vi "ABR-Init Level Series.vi"(0 "Stimulus":T3={"Ear"=enum."Left", "Start (dB)"=20, "Waveform"=enum."TONE PIP", "Stop (dB)"=80, "Frequency (kHz)"=16.0, "Step (dB)"=5, "Rep rate (/sec)"=30.0, "Alternate Polarity"=FALSE} {"Frequency (kHz)" format="%.2f"; "Start (dB)" step=5}, 1 "Data Folder":path, 5 "Runtime In":T1, 9 "Hidden":T2={"AI Samp Rate Hz"=25000.0, "AO Samp Rate Hz"=100000.0, "Duration (ms)"=5.0, "Ramp (ms)"=0.5, "Click width (us)"=0.0, "ITI"=enum."Rate", "Save raw"=FALSE}, 11 "error in (no error)":errorcluster) -> (6 "Runtime Out":T1, 15 "error out":errorcluster)   [LabVIEW 2020]
uses:
  TypeDefs/ABR-Stimulus.ctl
  TypeDefs/ABR-Hidden Params.ctl
  TypeDefs/ABR-Runtime Data.ctl
  epl-vi-lib/Signal Synthesis VIs/Waveform VIs/Pulse Train VIs/Pulse Train Params.ctl
  epl-vi-lib/Signal Synthesis VIs/Waveform VIs/Pulse Train VIs/Pulse Polarity.ctl
  epl-vi-lib/Signal Synthesis VIs/Waveform VIs/Pulse Train VIs/PT-Continuous State.ctl
  epl-vi-lib/Utility VIs/Type Defs/Speaker ring.ctl
panel:
  out "chan index":i32
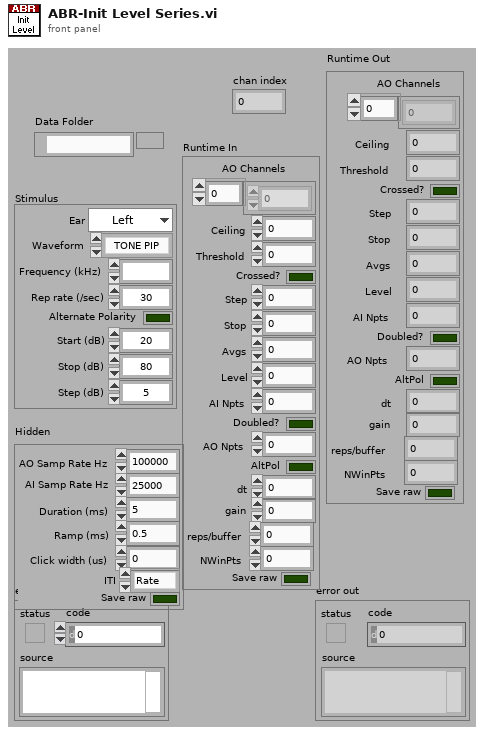
[diagram p1: front panel]
types:
  T1 = typedef "ABR-Runtime Data.ctl" = cluster{"AO Channels":i32[], "Ceiling":dbl, "Threshold":dbl, "Crossed?":bool, "Step":dbl, "Stop":i32, "Avgs":i32, "Level":dbl, "AI Npts":i32, "Doubled?":bool, "AO Npts":i32, "AltPol":bool, "dt":dbl, "gain":dbl, "reps/buffer":i32, "NWinPts":i32, "Save raw":bool}
  T2 = typedef "ABR-Hidden Params.ctl" = cluster{"AI Samp Rate Hz":dbl, "AO Samp Rate Hz":dbl, "Duration (ms)":dbl, "Ramp (ms)":dbl, "Click width (us)":dbl, "ITI":enum16{"Rate", "Interval"}, "Save raw":bool}
  T3 = typedef "ABR-Stimulus.ctl" = cluster{"Ear":enum16{"Right", "Left", "Bone"}, "Start (dB)":i32, "Waveform":enum16{"TONE PIP", "CLICK"}, "Stop (dB)":i32, "Frequency (kHz)":ext, "Step (dB)":i32, "Rep rate (/sec)":dbl, "Alternate Polarity":bool}
  T4 = typedef "Pulse Train Params.ctl" = cluster{"Pulse width (us)":dbl, "Pulse rate (Hz)":dbl, "Gap (ms)":dbl, "Polarity":T5, "PT State":T6, "Asynch":bool}
  T5 = typedef "Pulse Polarity.ctl" = enum16{"POS", "NEG", "POS-NEG", "NEG-POS"}
  T6 = typedef "PT-Continuous State.ctl" = cluster{"Template":dbl[], "Nperiod":i32, "Index":i32, "Pulse Rate (Hz)":dbl, "Phase (cycles)":dbl, "Noff":i32}
  T7 = typedef "Speaker ring.ctl" = enum16{"Right primary", "Right secondary", "Left primary", "Left secondary"}
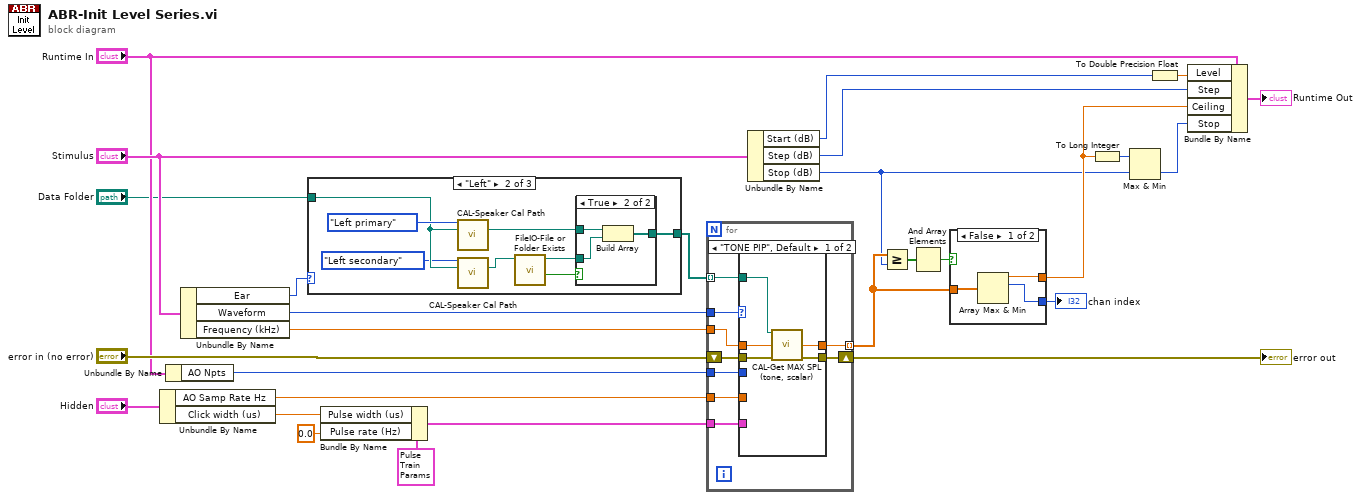
[diagram p0: block diagram]
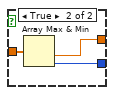
[diagram p2: hidden frame]
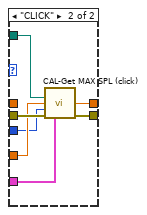
[diagram p3: hidden frame]
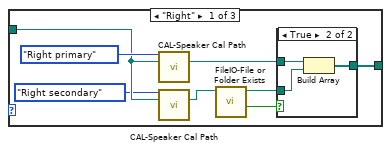
[diagram p4: hidden frame]
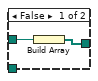
[diagram p5: hidden frame]
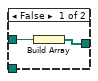
[diagram p6: hidden frame]
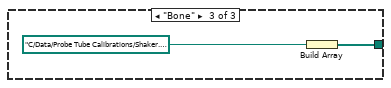
[diagram p7: hidden frame]
diagram:
  n1 = Unbundle By Name("Hidden") -> ("AO Samp Rate Hz"=w12:dbl, "Click width (us)"=w11:dbl)
  n2 = Unbundle By Name("Runtime In") -> ("AO Npts"=w9:i32)
  n3 = Unbundle By Name("Stimulus") -> ("Ear"=w24:enum16{"Right", "Left", "Bone"}, "Waveform"=w27:enum16{"TONE PIP", "CLICK"}, "Frequency (kHz)"=w26:ext)
  n4 = case shown="\"Left\"" w24 {
    tunnel: "Data Folder" -> [w35 w48 _]
    tunnel: [w32 w45 w55] -> w7
    frame "Right" {
      n5 = call "CAL-Speaker Cal Path.vi"("Speaker"=Speaker_ring."Right primary", "Data Folder"=w35) -> ("Cal Path"=w33:path)  [unwired: 12 in, 1 out]
      n6 = call "CAL-Speaker Cal Path.vi"("Speaker"=Speaker_ring."Right secondary", "Data Folder"=w35) -> ("Cal Path"=w31:path)  [unwired: 12 in, 1 out]
      n7 = call "FileIO-File or Folder Exists.vi"("path"=w31) -> ("Exists?"=w29:bool, "dup path"=w30:path)  [unwired: 7 in, 2 out]
      n8 = case shown="True" w29 {
        tunnel: w33 -> [w38 w41]
        tunnel: [w37 w40] -> w32
        tunnel: w30 -> [_ w39]
        frame False {
          n9 = Build Array(w38) -> (w37:path[])
        }
        frame True {
          n10 = Build Array(w41, w39) -> (w40:path[])
        }
      }
    }
    frame "Left" {
      n11 = call "CAL-Speaker Cal Path.vi"("Speaker"=Speaker_ring."Left primary", "Data Folder"=w48) -> ("Cal Path"=w46:path)  [unwired: 12 in, 1 out]
      n12 = call "CAL-Speaker Cal Path.vi"("Speaker"=Speaker_ring."Left secondary", "Data Folder"=w48) -> ("Cal Path"=w44:path)  [unwired: 12 in, 1 out]
      n13 = call "FileIO-File or Folder Exists.vi"("path"=w44) -> ("Exists?"=w42:bool, "dup path"=w43:path)  [unwired: 7 in, 2 out]
      n14 = case shown="True" w42 {
        tunnel: w46 -> [w51 w54]
        tunnel: [w50 w53] -> w45
        tunnel: w43 -> [_ w52]
        frame False {
          n15 = Build Array(w51) -> (w50:path[])
        }
        frame True {
          n16 = Build Array(w54, w52) -> (w53:path[])
        }
      }
    }
    frame "Bone" {
      n17 = Build Array(path "C:/Data/Probe Tube Calibrations/Shaker.calib" ("Cal Path")) -> (w55:path[])
    }
  }
  n18 = Bundle By Name(cluster=T4 {"Pulse width (us)"=0.0, "Pulse rate (Hz)"=0.0, "Gap (ms)"=0.0, "Polarity"=enum."POS", "PT State"={"Template"=[], "Nperiod"=0, "Index"=0, "Pulse Rate (Hz)"=0.0, "Phase (cycles)"=0.0, "Noff"=0}, "Asynch"=FALSE} ("Pulse Train Params"), "Pulse width (us)"=w11, "Pulse rate (Hz)"=0.0) -> (w20:T4)
  n19 = for {
    tunnel: w27 -> [w64]
    tunnel: w26 -> [w63]
    tunnel: w20 -> [w62]
    tunnel: w9 -> [w58]
    tunnel: w7 -> [w57] mode=indexing
    shift-right: [w61] -> w19
    shift-left: "error in (no error)" -> [w65]
    tunnel: w12 -> [w59]
    tunnel: [w60] -> w5 mode=indexing
    n20 = case shown="\"TONE PIP\", Default" w64 {
      tunnel: w65 -> [w70 w77]
      tunnel: w63 -> [w67 _]
      tunnel: [w69 w76] -> w61
      tunnel: [w68 w75] -> w60
      tunnel: w57 -> [w66 w74]
      tunnel: w62 -> [_ w73]
      tunnel: w59 -> [_ w72]
      tunnel: w58 -> [_ w71]
      frame "TONE PIP", Default {
        n21 = call "CAL-Get MAX SPL (tone, scalar).vi"("Cal Path"=w66, "Frequency (kHz)"=w67, "error in (no error)"=w70) -> ("Max SPL"=w68:dbl, "error out"=w69:errorcluster)  [unwired: 11 in]
      }
      frame "CLICK" {
        n22 = call "CAL-Get MAX SPL (click).vi"("Cal path"=w74, "Sampling Rate (Hz)"=w72, "Npts"=w71, "error in (no error)"=w77, "Pulse Train Params"=w73) -> ("Peak SPL"=w75:dbl, "error out"=w76:errorcluster)  [unwired: 9 in]
      }
    }
  }
  "error out" <- w19
  n23 = Unbundle By Name("Stimulus") -> ("Start (dB)"=w15:i32, "Step (dB)"=w13:i32, "Stop (dB)"=w4:i32)
  n24 = Greater Or Equal?(x=w5, y=w4) -> (x >= y?=w3:bool[])
  n25 = And Array Elements(Boolean array=w3) -> (logical AND=w2:bool)
  n26 = case shown="False" w2 {
    tunnel: [w80 w82] -> w6
    tunnel: w5 -> [w79 w83]
    tunnel: [w78 w81] -> w1
    frame False {
      n27 = Array Max & Min(array=w79) -> (max value=w80:dbl, max index (indices)=w78:i32)  [unwired: 2 out]
    }
    frame True {
      n28 = Array Max & Min(array=w83) -> (min value=w82:dbl, min index (indices)=w81:i32)  [unwired: 2 out]
    }
  }
  "chan index" <- w1
  n29 = To Long Integer(number=w6) -> (32bit integer=w17:i32)
  n30 = Max & Min(x=w17, y=w4) -> (min(x,y)=w14:i32)  [unwired: 1 out]
  n31 = To Double Precision Float(number=w15) -> (double precision float=w18:dbl)
  n32 = Bundle By Name(cluster="Runtime In", "Level"=w18, "Step"=w13, "Ceiling"=w6, "Stop"=w14) -> (→"Runtime Out":T1)
